vi "sv_Resample (Const to Variable, DBL Array) with IC.vi"(0 "Array":dbl[](array[numeric]) format="%.2f", 1 "sampling rate":dbl=1.0, 3 "reset? (True)":bool=TRUE, 5 "time":dbl[](array[numeric]) format="%.2f", 9 "filter prototype":T2={"left wing"=[], "increment"=[], "max dec"=128, "timing jitter"=enum."Interpolation", "band limiting?"=TRUE} {"increment" format="%.2f"; "left wing" format="%.2f"}, 11 "initial conditions":T1, 12 "channel count":i32) -> (4 "Y":dbl[][](array[numeric]) format="%.2f", 6 "time stamps":dbl[](array[numeric]) format="%.2f", 10 "offset":dbl, 15 "final conditions":T1)   [LabVIEW 2017, in "SoundVib_Resampling.lvlib"]
doc: "Perform an arbitrary resampling on the input signal."
uses:
  <vilib>/addons/Sound and Vibration/Order Analysis/Resample Order Tracking/SoundVib_Resampling.lvlib
  <vilib>/addons/_NISVFA/_Shared subVIs/Controls/OAT Resample Filter Prototype.ctl
  <resource>/sndvib.dll
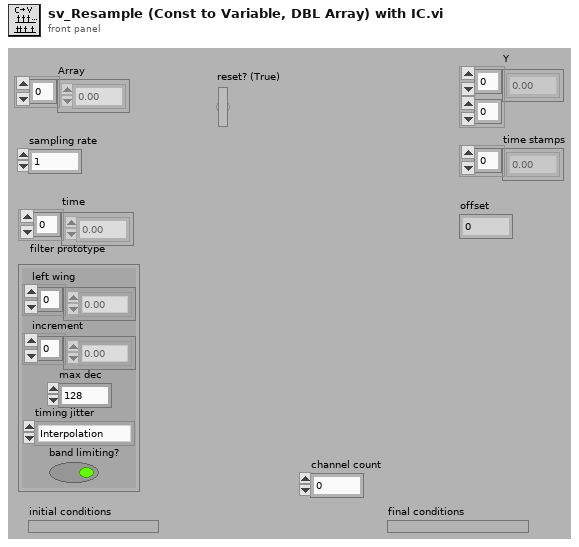
[diagram p1: front panel]
types:
  T1 = cluster{"signal length":u64, "time":dbl[], "reset state":bool, "state":cluster{"init condition":dbl[], "start index":i32, "channel count":i32, "condition len":i32, "position":dbl, "time interval":dbl, "max cond len":i32}, "offset":dbl}
  T2 = typedef "OAT Resample Filter Prototype.ctl" = cluster{"left wing":dbl[], "increment":dbl[], "max dec":i32, "timing jitter":enum32{"Interpolation", "Rounding"}, "band limiting?":bool}
  T3 = cluster{"init condition":dbl[], "start index":i32, "channel count":i32, "condition len":i32, "position":dbl, "time interval":dbl, "max cond len":i32}
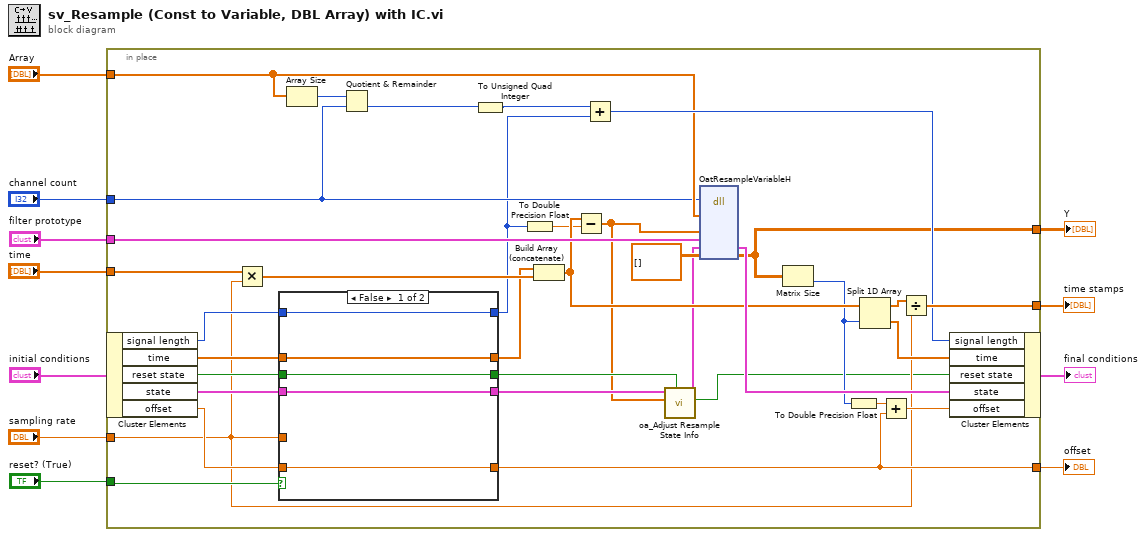
[diagram p0: block diagram]
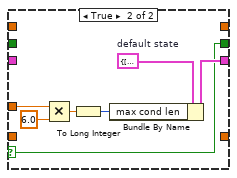
[diagram p2: hidden frame]
diagram:
  n1 = in-place {
    in-place-border: "filter prototype" -> [w46]
    in-place-border: "time" -> [w45]
    in-place-border: [w18] -> w9
    in-place-border: [w44] -> w8
    in-place-border: [w43] -> w7
    in-place-border: "channel count" -> [w23]
    in-place-border: "sampling rate" -> [w27]
    in-place-border: "Array" -> [w24]
    in-place-border: "reset? (True)" -> [w29]
    n2 = in-place-cluster #1("initial conditions") -> ("signal length"=w40:u64, "time"=w39:dbl[], "reset state"=w28:bool, "state"=w38:T3, "offset"=w34:dbl)
    n3 = Multiply(x=w45, y=w27) -> (x*y=w41:dbl[])
    n4 = case shown="False" w29 {
      selector: w29 -> [_ w52]
      tunnel: [w51 _] -> w44
      tunnel: w40 -> [w48 _]
      tunnel: w39 -> [w49 _]
      tunnel: w38 -> [w50 _]
      tunnel: w34 -> [w51 _]
      tunnel: [w49 _] -> w32
      tunnel: [w48 _] -> w20
      tunnel: [w50 w58] -> w15
      tunnel: [w47 w52] -> w16
      tunnel: w28 -> [w47 _]
      tunnel: w27 -> [_ w54]
      frame False {
      }
      frame True {
        w53 = T3 {"init condition"=[], "start index"=0, "channel count"=0, "condition len"=0, "position"=0.0, "time interval"=0.0, "max cond len"=0}  # default state
        n5 = Multiply(x=w54, y=6.0) -> (x*y=w57:dbl)
        n6 = To Long Integer(number=w57) -> (32bit integer=w55:i32)
        n7 = Bundle By Name(cluster=w53, "max cond len"=w55) -> (w58:T3)
      }
    }
    n8 = Array Size(array=w24) -> (size(s)=w25:i32)
    n9 = Quotient & Remainder(x=w25, y=w23) -> (floor(x/y)=w22:i32)  [unwired: 1 out]
    n10 = To Unsigned Quad Integer(1:w22) -> (0:w21:u64)
    n11 = To Double Precision Float(number=w20) -> (double precision float=w19:dbl)
    n12 = Build Array (concatenate)(w32, w41) -> (w31:dbl[])
    n13 = Subtract(x=w31, y=w19) -> (x-y=w12:dbl[])
    n14 = Add(x=w21, y=w20) -> (x+y=w37:u64)
    n15 = call <vilib>:"oa_Adjust Resample State Info.vi"("Reset? (True)"=w16, "time position"=w12, "state in"=w15) -> ("reset pending"=w13:bool, "state out"=w14:T3)  [unwired: 7 in]
    n16 = dll-call lib="C:/Program Files (x86)/National Instruments/LabVIEW 2017/resource/sndvib.*" fn="OatResampleVariableH"("signalH"=w24, "channelCount"=w23, "timeH"=w12, "prototype"=w46, "state"=w14, "yH"=dbl[][] []) -> ("state"=w35:T3, "yH"=w18:dbl[][])  [unwired: 8 in, 2 out]
    n17 = Matrix Size(0:w18) -> (2:w17:i32)  [unwired: 1 out]
    n18 = To Double Precision Float(number=w17) -> (double precision float=w26:dbl)
    n19 = Split 1D Array(array=w31, index=w17) -> (first subarray=w42:dbl[], second subarray=w36:dbl[])
    n20 = Add(x=w26, y=w44) -> (x+y=w33:dbl)
    n21 = Divide(x=w42, y=w27) -> (x/y=w43:dbl[])
    n22 = in-place-cluster #1("signal length"=w37, "time"=w36, "reset state"=w13, "state"=w35, "offset"=w33) -> (→"final conditions":T1)
  }
  "time stamps" <- w7
  "Y" <- w9
  "offset" <- w8
